vi "Wojtek Controller.vi"(8 "kp":dbl=0.02, 9 "kd":dbl=0.0015, 10 "Current Angle":dbl[](array[numeric])=[-1.0340072183364002, 0.012772422572544642], 11 "Speed":dbl format="%#_13g") -> (2 "left axis value":dbl=-0.5206609857328692, 3 "right axis value":dbl=-0.4793390142671308)   [LabVIEW 2014]
doc: "This VI uses a PD controller to keep the robot straight during Autonomous Mode."
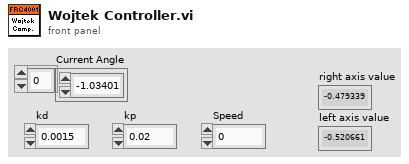
[diagram p1: front panel]
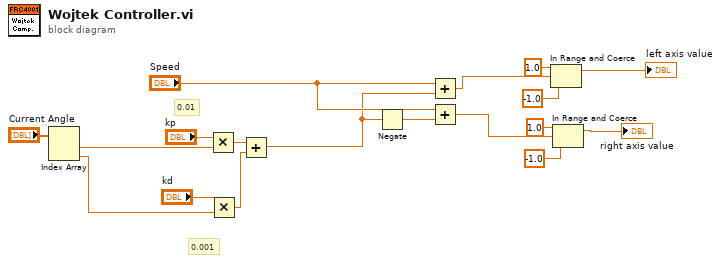
[diagram p0: block diagram]
diagram:
  # "0.01"
  # "0.001"
  n1 = Index Array(array="Current Angle") -> (element #1=w14:dbl, element #2=w13:dbl)  [unwired: 2 in]
  n2 = Multiply(x="kp", y=w14) -> (x*y=w18:dbl)
  n3 = Multiply(x="kd", y=w13) -> (x*y=w17:dbl)
  n4 = Add(x=w18, y=w17) -> (x+y=w2:dbl)
  n5 = Negate(x=w2) -> (-x=w1:dbl)
  n6 = Add(x="Speed", y=w2) -> (x+y=w8:dbl)
  n7 = Add(x="Speed", y=w1) -> (x+y=w12:dbl)
  n8 = In Range and Coerce(upper limit=1.0, x=w8, lower limit=-1.0) -> (coerced(x)=→"left axis value":dbl)  [unwired: 1 out]
  n9 = In Range and Coerce(upper limit=1.0, x=w12, lower limit=-1.0) -> (coerced(x)=→"right axis value":dbl)  [unwired: 1 out]
